vi "Merge.vi"(8 "error in (no error)":errorcluster, 10 "Field To Merge":refnum<class "Field.lvclass">, 11 "FK Ring In":refnum<class "FK Ring.lvclass">) -> (0 "error out":errorcluster, 3 "Merged FK Ring out":refnum<class "FK Ring.lvclass">)   [LabVIEW 2020, in "FK Ring.lvclass"]
uses:
  FK Ring.lvclass
  Field/Field.lvclass
  FK Ring.lvclass/FK Ring.ctl
  Ring Field/Ring Field.lvclass
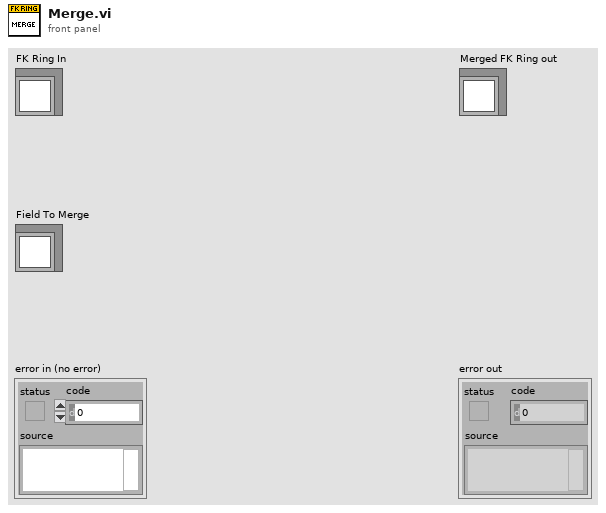
[diagram p1: front panel]
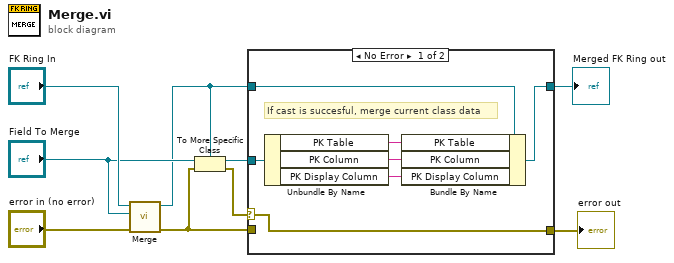
[diagram p0: block diagram]
diagram:
  n1 = call-parent "Merge.vi"("error in (no error)"="error in (no error)", "Field To Merge"="Field To Merge", "Field In"="FK Ring In") -> ("error out"=w1:errorcluster, "Merged Field out"=w4:refnum<class "FK Ring.lvclass">)  [unwired: 7 in]
  n2 = To More Specific Class(target class=w4, reference="Field To Merge", error in=w1) -> (specific class reference=w3:refnum<class "FK Ring.lvclass">, error out=w2:errorcluster)
  n3 = case shown="No Error" w2 {
    selector: w2 -> [w10 _]
    tunnel: w4 -> [w15 w18]
    tunnel: [w14 w18] -> w7
    tunnel: [w10 w17] -> w6
    tunnel: w3 -> [w16 _]
    tunnel: w1 -> [_ w17]
    frame No Error {
      # "If cast is succesful, merge current class data"
      n4 = Unbundle By Name(w16) -> ("PK Table"=w13:string, "PK Column"=w12:string, "PK Display Column"=w11:string)
      n5 = Bundle By Name(cluster=w15, "PK Table"=w13, "PK Column"=w12, "PK Display Column"=w11) -> (w14:refnum<class "FK Ring.lvclass">)
    }
    frame Error {
      # "If an error happens or the downcast fails, meaning\nthere is no additional member data to merge,\nreturn parent's error"
    }
  }
  "error out" <- w6
  "Merged FK Ring out" <- w7
